vi "GenerateHtmlDoc.vi"(8 "error in":errorcluster, 10 "Clear":bool, 11 "Vi":path) -> (0 "error out":errorcluster, 1 "Title":string, 2 "VI Description":string, 3 "Html Path":path)   [LabVIEW 2020]
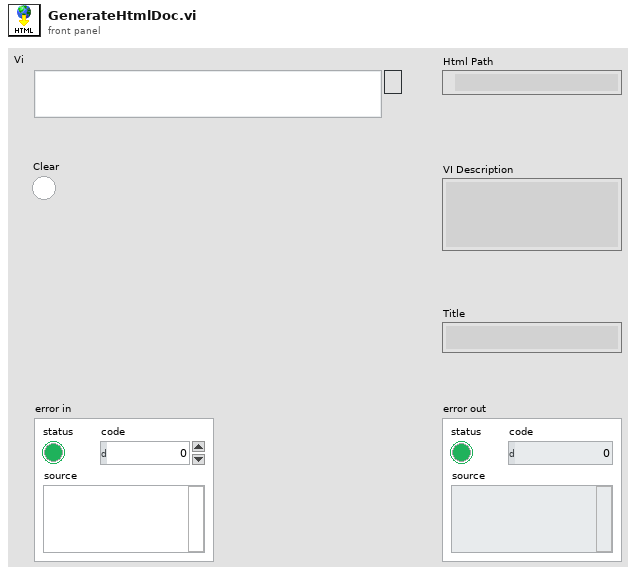
[diagram p1: front panel]
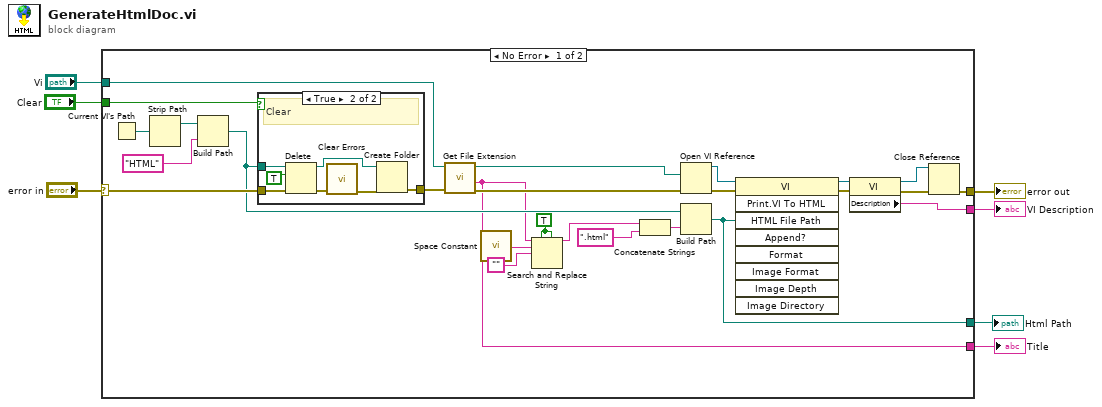
[diagram p0: block diagram]
diagram:
  n1 = case shown="No Error" "error in" {
    selector: "error in" -> [w20 w42]
    tunnel: "Vi" -> [w27 _]
    tunnel: [w22 w42] -> w6
    tunnel: [w21 _] -> w5
    tunnel: [w15 _] -> w3
    tunnel: "Clear" -> [w14 _]
    tunnel: [w8 _] -> w1
    frame No Error {
      w10 = TRUE
      n2 = Current VI's Path() -> (path=w33:path)
      n3 = Strip Path(path=w33) -> (stripped path=w32:path)  [unwired: 1 out]
      n4 = Build Path(base path=w32, name or relative path="HTML") -> (appended path=w13:path)
      n5 = case shown="True" w14 {
        tunnel: w13 -> [_ w41]
        tunnel: [w34 w37] -> w28
        tunnel: w20 -> [w34 w36]
        frame False {
        }
        frame True {
          # "Clear"
          n6 = Delete(path (use dialog)=w41, entire hierarchy (F)=TRUE, error in=w36) -> (deleted path=w39:path, error out=w40:errorcluster)  [unwired: 2 in, 1 out]
          n7 = call <vilib>:"Clear Errors.vi"("error in (no error)"=w40) -> ("error out"=w38:errorcluster)  [unwired: 5 in, 1 out]
          n8 = Create Folder(path (use dialog)=w39, error in=w38) -> (error out=w37:errorcluster)  [unwired: 1 in, 2 out]
        }
      }
      n9 = call <vilib>:"Get File Extension.vi"("error in (no error)"=w28, "file"=w27) -> ("error out"=w25:errorcluster, "filename without extension"=w8:string, "dup file"=w26:path)  [unwired: 5 in, 2 out]
      n10 = call <vilib>:"Space Constant.vi"() -> ("String"=w12:string)
      n11 = Search and Replace String(replace all?=w10, case sensitive?=w10, input string=w8, search string=w12, replace string="") -> (result string=w9:string)  [unwired: 3 in, 3 out]
      n12 = Concatenate Strings(w9, ".html") -> (w24:string)
      n13 = Open VI Reference(vi path=w26, error in (no error)=w25) -> (vi reference=w29:refnum<vi>, error out=w30:errorcluster)  [unwired: 4 in]
      n14 = Build Path(base path=w13, name or relative path=w24) -> (appended path=w21:path)
      n15 = invoke class="VI" method="Print.VI To HTML"(reference=w29, error in=w30, "HTML File Path"=w21) -> (reference out=w19:refnum<vi>, error out=w18:errorcluster)  [unwired: 6 in, 7 out]
      n16 = property class="VI"(reference=w19, error in=w18) -> (reference out=w17:refnum<vi>, error out=w16:errorcluster, "Description"=w15:string)
      n17 = Close Reference(reference=w17, error in (no error)=w16) -> (error out=w22:errorcluster)
    }
    frame Error {
    }
  }
  "Html Path" <- w5
  "error out" <- w6
  "VI Description" <- w3
  "Title" <- w1
